vi "Control Loop.vi"   [LabVIEW 2009]
uses:
  TypeDefs/State Machine/Main State.ctl
  <vilib>/Platform/TimedLoop/XDataNode/XDataNode.xnode
  <vilib>/Platform/TimedLoop/XDataNode/loadlvalarms.vi
  <vilib>/Platform/TimedLoop/XDataNode/timing_clust.ctl
  <vilib>/Platform/TimedLoop/XDataNode/nitl_modes.ctl
  <vilib>/Platform/TimedLoop/XDataNode/wakeup.ctl
  Functional Global Variables/Actions for FG's.ctl
  TypeDefs/Queue TypeDefs/Motor Instruction.ctl
  TypeDefs/Queue TypeDefs/Motor State.ctl
  Remote Control/Motor Command.ctl
  <vilib>/userDefined/High Color/nirio_resource_hc.ctl
  <vilib>/rvi/interface/nirviOpenFPGA/nirviOpenFPGA.xnode
  FPGA Bitfiles/Q_IGVC_2010.lvproj_FPGA Target_FPGA_MAIN.vi.lvbitx
  <vilib>/FPGAPlugInAG/cRIO-9113/nirviIntfOpen_cRIO-9113.vi
  <vilib>/Platform/TimedLoop/XDataNode/XDNodeRunTimeDep.lvlib
  <vilib>/NI_Real-Time Target Support.lvlib
types:
  T1 = typedef "Main State.ctl" = enum16{"Startup", "Wait for Init", "Initialize Sensors", "Wait for Saftey Disable", "Check Saftey", "Wait for GO", "Run", "Remote Control", "Stop"}
  T2 = typedef "XDNodeRunTimeDep.lvlib/timing_clust.ctl" = cluster{"Expected End [f-1]":u64, "Actual End [f-1]":u64, "Finished Late? [f-1]":bool, "Expected End [i-1]":u64, "Actual End [i-1]":u64, "Finished Late? [i-1]":bool, "Expected Start [i]":u64, "Actual Start [i]":u64, "Expected Start [f]":u64, "Actual Start [f]":u64, "Source Name":string, "Structure Name":string, "Period":i64, "Deadline":i64, "Offset":i64, "Start":i64, "Priority":i32, "Timeout":i32, "Mode":T3, "Wakeup Reason":T4, "Error":errorcluster, "Source Type":string, "Secondary Source Type":string, "Global End Time":u64, "Global Start Time":u64, "Frame Duration":u64, "Iteration Duration":u64, "Assigned CPU":i32, "I/O Scan Engine Mode":u32}
  T3 = typedef "XDNodeRunTimeDep.lvlib/nitl_modes.ctl" = enum32{"No Change", "Process missed periods, maintain original phase", "Discard missed periods, maintain original phase", "Process missed periods, ignore original phase", "Discard missed periods, ignore original phase"}
  T4 = typedef "XDNodeRunTimeDep.lvlib/wakeup.ctl" = enum32{"Normal", "Aborted", "Asynchronous wakeup", "Timing source error", "Timed loop error", "Timeout"}
  T5 = typedef "Actions for FG's.ctl" = enum16{"Read", "Write"}
  T6 = typedef "nirio_resource_hc.ctl" = tag
  T7 = cluster{"signature":u8[], "vi signatures match":bool, "signature register address":u32, "reset register address":u32, "control register address":u32, "interrupt base address":u32, "Bitstream Version":u32, "DMA Configuration":cluster{"Name":string, "Depth":u32, "Write? (Deprecated:Use Implementation)":bool, "Physical Channel":u32, "Base Address":u32, "Data Width":u32, "Data Type":enum32{"Boolean", "I8", "I16", "I32", "I64", "U8", "U16", "U32", "U64", "FXP"}, "FXP Properties":variant, "Write Window Address":u32, "Implementation":enum16{"niFpgaTargetToHost", "niFpgaHostToTarget", "niFpgaPeerToPeerWriter", "niFpgaPeerToPeerReader", "niCoreTargetToHost", "niCoreHostToTarget"}, "Control Set":u32}[], "run when loaded?":bool, "reset register size in bits":u32, "compilation results xml":string}
  T8 = typedef "Motor State.ctl" = enum16{"Wait", "Initialize", "Check FET", "Run", "Stop"}
  T9 = typedef "Motor Instruction.ctl" = cluster{"Motor State":T8, "Motor Command":T10}
  T10 = typedef "Motor Command.ctl" = cluster{"Speed":i16, "Turn":i16}
  T11 = typedef "FPGA Main ref.ctl" = refnum<k20>
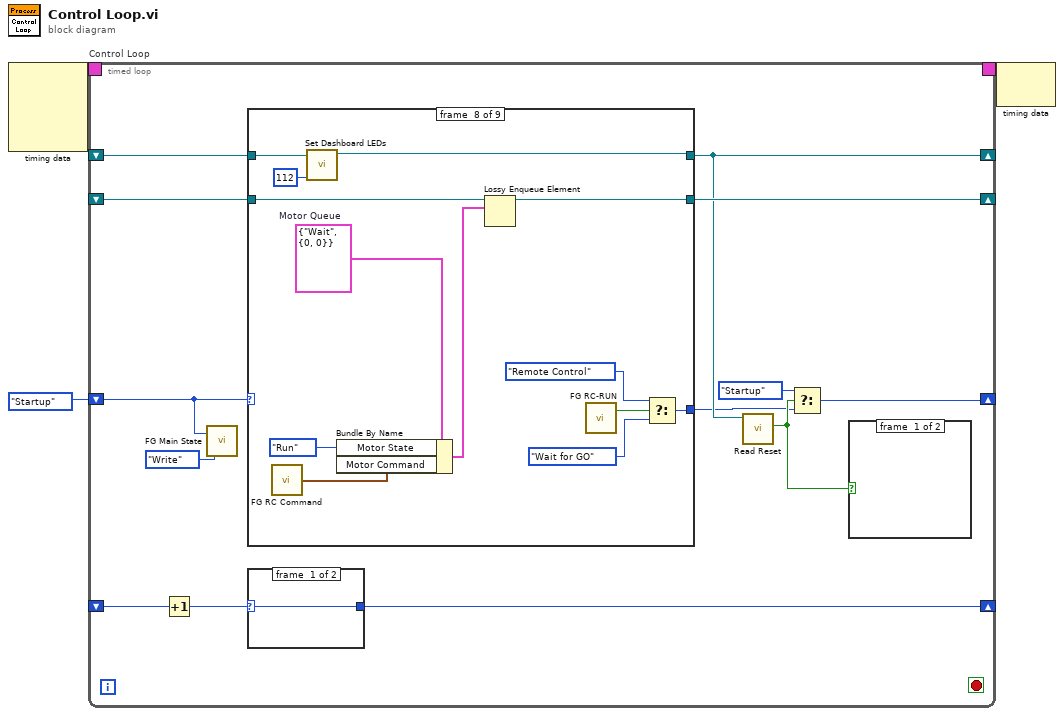
[diagram p0: block diagram]
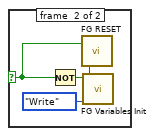
[diagram p2: hidden frame]
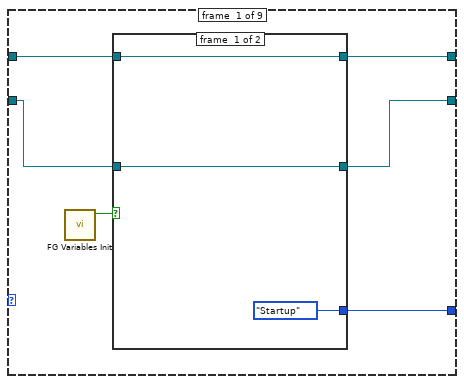
[diagram p3: hidden frame]
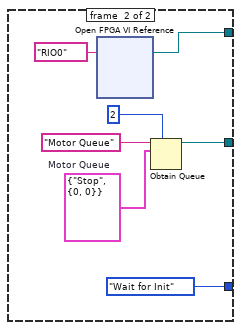
[diagram p4: hidden frame]
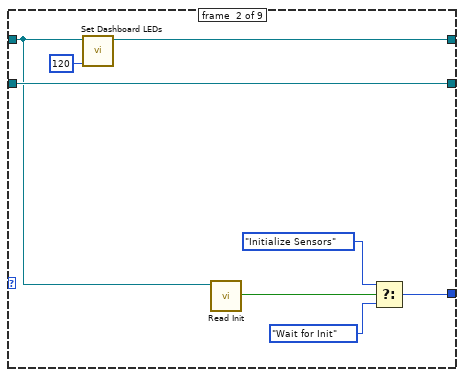
[diagram p5: hidden frame]
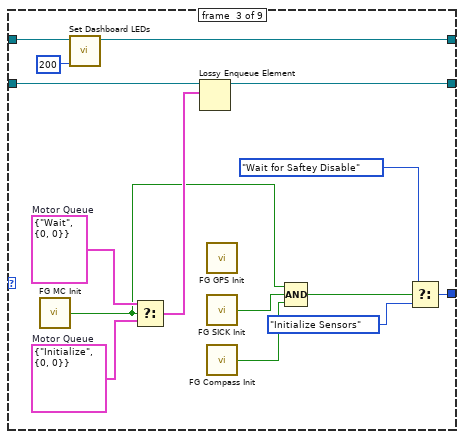
[diagram p6: hidden frame]
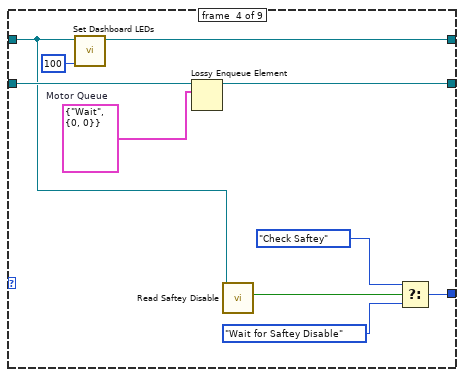
[diagram p7: hidden frame]
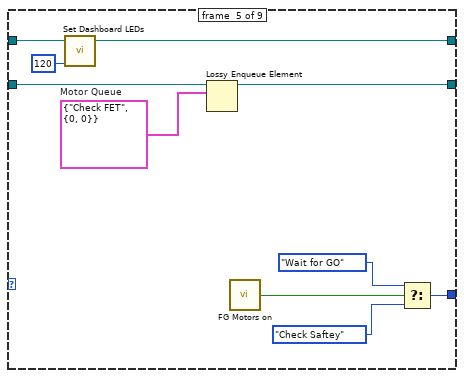
[diagram p8: hidden frame]
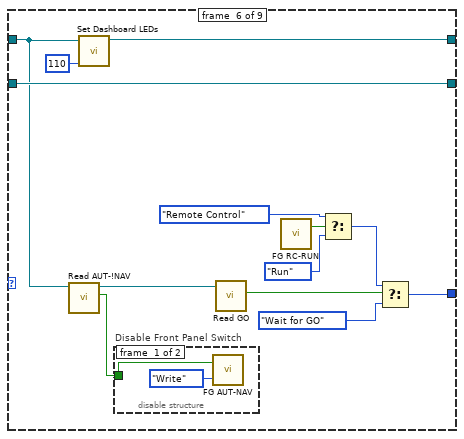
[diagram p9: hidden frame]
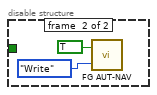
[diagram p10: hidden frame]
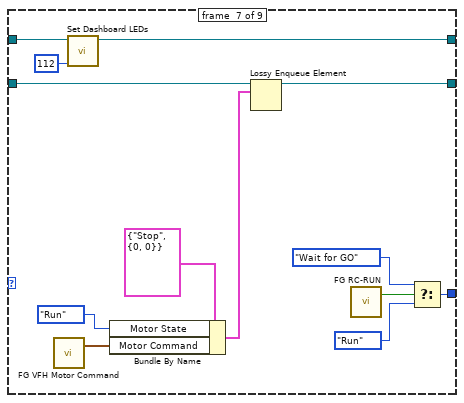
[diagram p11: hidden frame]
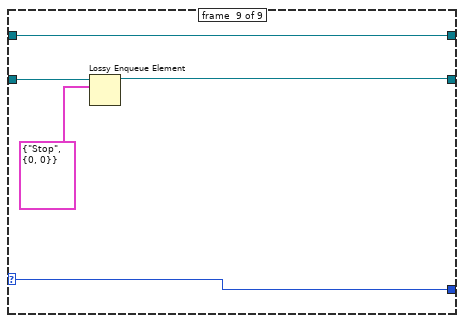
[diagram p12: hidden frame]
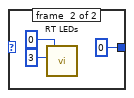
[diagram p13: hidden frame]
diagram:
  n1 = node-c288() -> (w3:T2)  [unwired: 4 in]
  n2 = timed-loop "Control Loop" {
    timing: w3 -> [_]
    timing-out: [_] -> w2
    shift-right: [w14] -> _
    shift-left: _ -> [w16]
    shift-right: [w9] -> _
    shift-left: Main_State."Startup" ("Main State") -> [w12]
    shift-right: [w10] -> _
    shift-left: _ -> [w13]
    shift-right: [w7] -> _
    shift-left: _ -> [w6]
    stop <- _ stop-if-true
    n3 = Increment(x=w16) -> (x+1=w15:i32)
    n4 = call "FG Main State.vi"("FG Action"=Actions_for_FG's."Write", "Main State in"=w12) -> ()  [unwired: 1 out]
    n5 = case shown="\"Wait for GO\"" w12 {
      selector: w12 -> [_ _ _ _ _ _ _ _ w134]
      tunnel: w6 -> [w20 w48 w56 w71 w81 w91 w110 w125 w133]
      tunnel: w13 -> [w22 w49 w69 w79 w88 w92 w114 w132 w137]
      tunnel: [w21 w50 w62 w73 w83 w95 w113 w126 w134] -> w5
      tunnel: [w24 w49 w57 w72 w82 w92 w112 w121 w135] -> w10
      tunnel: [w23 w47 w55 w70 w80 w90 w111 w120 w133] -> w7
      frame #0 {
        n6 = call "FG Variables Init.vi"() -> ("Variables Init out"=w25:bool)  [unwired: 11 in]
        n7 = case shown="True" w25 {
          tunnel: [w26 w34] -> w23
          tunnel: [w28 w30] -> w24
          tunnel: w22 -> [w28 _]
          tunnel: [Main_State."Startup" ("Main State") Main_State."Wait for Init" ("Main State")] -> w21
          tunnel: w20 -> [w26 _]
          frame #0 {
          }
          frame #1 {
            w32 = T9 {"Motor State"=enum."Stop", "Motor Command"={"Speed"=0, "Turn"=0}}  # Motor Queue
            n8 = xnode "Open FPGA VI Reference"("resource name"=T6 "RIO0") -> ("FPGA VI Reference Out"=w34:refnum<k20>)  [unwired: 1 in, 1 out]
            n9 = Obtain Queue(max queue size (-1, unlimited)=2, name (unnamed)="Motor Queue", element data type=w32) -> (queue out=w30:refnum<queue>)  [unwired: 2 in, 2 out]
          }
        }
      }
      frame #1 {
        n10 = call "Set Dashboard LEDs.vi"("Display code"=u8 120, "FPGA VI Reference in"=w48) -> ("FPGA VI Reference out"=w47:T11)  [unwired: 9 in]
        n11 = call "Read Init.vi"("FPGA VI Reference in"=w48) -> ("Init switch"=w54:bool)  [unwired: 7 in, 2 out]
        n12 = Select(t=Main_State."Initialize Sensors" ("Main State out"), s=w54, f=Main_State."Wait for Init" ("Main State out")) -> (s? t:f=w50:T1)
      }
      frame #2 {
        w60 = T9 {"Motor State"=enum."Initialize", "Motor Command"={"Speed"=0, "Turn"=0}}  # Motor Queue
        w61 = T9 {"Motor State"=enum."Wait", "Motor Command"={"Speed"=0, "Turn"=0}}  # Motor Queue
        n13 = call "FG MC Init.vi"() -> ("MC Init out"=w58:bool)  [unwired: 2 in]
        n14 = call "Set Dashboard LEDs.vi"("Display code"=u8 200, "FPGA VI Reference in"=w56) -> ("FPGA VI Reference out"=w55:T11)  [unwired: 9 in]
        n15 = Select(t=w61, s=w58, f=w60) -> (s? t:f=w59:T9)
        n16 = Lossy Enqueue Element(queue=w69, element=w59) -> (queue out=w57:refnum<queue>)  [unwired: 1 in, 3 out]
        n17 = call "FG GPS Init.vi"() -> ()  [unwired: 2 in, 1 out]
        n18 = call "FG SICK Init.vi"() -> ("SICK Init out"=w68:bool)  [unwired: 2 in]
        n19 = call "FG Compass Init.vi"() -> ("Compass Init out"=w67:bool)  [unwired: 2 in]
        n20 = Compound Arithmetic op=AND(w58, w68, w67) -> (w66:bool)
        n21 = Select(t=Main_State."Wait for Saftey Disable" ("Main State out"), s=w66, f=Main_State."Initialize Sensors" ("Main State out")) -> (s? t:f=w62:T1)
      }
      frame #3 {
        w78 = T9 {"Motor State"=enum."Wait", "Motor Command"={"Speed"=0, "Turn"=0}}  # Motor Queue
        n22 = call "Set Dashboard LEDs.vi"("Display code"=u8 100, "FPGA VI Reference in"=w71) -> ("FPGA VI Reference out"=w70:T11)  [unwired: 9 in]
        n23 = Lossy Enqueue Element(queue=w79, element=w78) -> (queue out=w72:refnum<queue>)  [unwired: 1 in, 3 out]
        n24 = call "Read Saftey Disable.vi"("FPGA VI Reference in"=w71) -> ("GO"=w74:bool)  [unwired: 7 in, 2 out]
        n25 = Select(t=Main_State."Check Saftey" ("Main State out"), s=w74, f=Main_State."Wait for Saftey Disable" ("Main State out")) -> (s? t:f=w73:T1)
      }
      frame #4 {
        w89 = T9 {"Motor State"=enum."Check FET", "Motor Command"={"Speed"=0, "Turn"=0}}  # Motor Queue
        n26 = call "Set Dashboard LEDs.vi"("Display code"=u8 120, "FPGA VI Reference in"=w81) -> ("FPGA VI Reference out"=w80:T11)  [unwired: 9 in]
        n27 = Lossy Enqueue Element(queue=w88, element=w89) -> (queue out=w82:refnum<queue>)  [unwired: 1 in, 3 out]
        n28 = call "FG Motors on.vi"() -> ("Motors on ? out"=w85:bool)  [unwired: 2 in]
        n29 = Select(t=Main_State."Wait for GO" ("Main State out"), s=w85, f=Main_State."Check Saftey" ("Main State out")) -> (s? t:f=w83:T1)
      }
      frame #5 {
        n30 = call "Read AUT-!NAV.vi"("FPGA VI Reference in"=w91) -> ("FPGA VI Reference out"=w93:T11, "AUT/!NAV"=w94:bool)  [unwired: 7 in, 1 out]
        n31 = call "Set Dashboard LEDs.vi"("Display code"=u8 110, "FPGA VI Reference in"=w91) -> ("FPGA VI Reference out"=w90:T11)  [unwired: 9 in]
        n32 = disable-structure "Disable Front Panel Switch" shown="Enabled" {
          disable-tunnel: w94 -> [w104 _]
          frame #0 {
            n33 = call "FG AUT-NAV.vi"("FG Action (Read)"=Actions_for_FG's."Write", "Aut/!Nav in"=w104) -> ()  [unwired: 1 out]
          }
          frame #1 {
            n34 = call "FG AUT-NAV.vi"("FG Action (Read)"=Actions_for_FG's."Write", "Aut/!Nav in"=TRUE) -> ()  [unwired: 1 out]
          }
        }
        n35 = call "Read GO.vi"("FPGA VI Reference in"=w93) -> ("GO"=w99:bool)  [unwired: 7 in, 2 out]
        n36 = call "FG RC-RUN.vi"() -> ("RC/!Run out"=w100:bool)  [unwired: 3 in]
        n37 = Select(t=Main_State."Remote Control" ("Main State"), s=w100, f=Main_State."Run" ("Main State")) -> (s? t:f=w97:T1)
        n38 = Select(t=w97, s=w99, f=Main_State."Wait for GO" ("Main State")) -> (s? t:f=w95:T1)
      }
      frame #6 {
        n39 = call "FG VFH Motor Command.vi"() -> ("Motor Command out"=w116:T10)  [unwired: 3 in]
        n40 = call "Set Dashboard LEDs.vi"("Display code"=u8 112, "FPGA VI Reference in"=w110) -> ("FPGA VI Reference out"=w111:T11)  [unwired: 9 in]
        n41 = Bundle By Name(cluster=T9 {"Motor State"=enum."Stop", "Motor Command"={"Speed"=0, "Turn"=0}} ("element"), "Motor State"=Motor_State."Run", "Motor Command"=w116) -> (w115:T9)
        n42 = Lossy Enqueue Element(queue=w114, element=w115) -> (queue out=w112:refnum<queue>)  [unwired: 1 in, 3 out]
        n43 = call "FG RC-RUN.vi"() -> ("RC/!Run out"=w107:bool)  [unwired: 3 in]
        n44 = Select(t=Main_State."Wait for GO" ("Main State"), s=w107, f=Main_State."Run" ("Main State")) -> (s? t:f=w113:T1)
      }
      frame #7 {
        w131 = T9 {"Motor State"=enum."Wait", "Motor Command"={"Speed"=0, "Turn"=0}}  # Motor Queue
        n45 = call "FG RC Command.vi"() -> ("Motor Command out"=w123:T10)  [unwired: 2 in]
        n46 = call "Set Dashboard LEDs.vi"("Display code"=u8 112, "FPGA VI Reference in"=w125) -> ("FPGA VI Reference out"=w120:T11)  [unwired: 9 in]
        n47 = Bundle By Name(cluster=w131, "Motor State"=Motor_State."Run", "Motor Command"=w123) -> (w122:T9)
        n48 = Lossy Enqueue Element(queue=w132, element=w122) -> (queue out=w121:refnum<queue>)  [unwired: 1 in, 3 out]
        n49 = call "FG RC-RUN.vi"() -> ("RC/!Run out"=w128:bool)  [unwired: 3 in]
        n50 = Select(t=Main_State."Remote Control" ("Main State"), s=w128, f=Main_State."Wait for GO" ("Main State")) -> (s? t:f=w126:T1)
      }
      frame #8 {
        n51 = Lossy Enqueue Element(queue=w137, element=T9 {"Motor State"=enum."Stop", "Motor Command"={"Speed"=0, "Turn"=0}}) -> (queue out=w135:refnum<queue>)  [unwired: 1 in, 3 out]
      }
    }
    n52 = case shown="10" w15 {
      selector: w15 -> [w138 _]
      tunnel: [w138 0] -> w14
      frame #0 {
      }
      frame #1 {
        n53 = call <vilib>:"RT LEDs.vi"("State"=3, "LED Num"=0) -> ()  [unwired: 4 in, 2 out]
      }
    }
    n54 = call "Read Reset.vi"("FPGA VI Reference in"=w7) -> ("Reset"=w8:bool)  [unwired: 8 in, 2 out]
    n55 = Select(t=Main_State."Startup", s=w8, f=w5) -> (s? t:f=w9:T1)
    n56 = case shown="True" w8 {
      selector: w8 -> [_ w17]
      frame #0 {
      }
      frame #1 {
        w18 = Actions_for_FG's."Write" ("FG Action (Read)")
        n57 = Not(x=w17) -> (.not. x?=w19:bool)
        n58 = call "FG RESET.vi"("FG Action (Read)"=w18, "RESET in"=w17) -> ()  [unwired: 1 out]
        n59 = call "FG Variables Init.vi"("FG Action"=w18, "Variables Init in"=w19) -> ()  [unwired: 9 in, 1 out]
      }
    }
  }
  n60 = node-c288(w2) -> ()  [unwired: 1 out]
